vi "Page_Source_Initialize.vi"(8 "error in (no error)":errorcluster, 9 "ctlReferences":T1, 11 "AB_PackedLibrary in":refnum<class "AB_PackedLibrary.lvclass">) -> (0 "error out":errorcluster, 1 "supportedFunctions":T2, 3 "AB_PackedLibrary out":refnum<class "AB_PackedLibrary.lvclass">)   [LabVIEW 2020, in "AB_PackedLibrary.lvclass"]
uses:
  <vilib>/AppBuilder/AB_Classes/PackedLib/AB_PackedLibrary.lvclass
  <resource>/Framework/Providers/Builds/AppBuilder/AB_UI_Page_Source_Files_supportedFunctions.ctl
  <vilib>/AppBuilder/AB_Source_Inclusion.ctl
  <resource>/Framework/Providers/Builds/AppBuilder/AB_UI_Page_Source_Files_References.ctl
  <resource>/Framework/Providers/Common/provcom_StringGlobals.vi
  <vilib>/AppBuilder/AB_Classes/TargetFile/AB_Targetfile.lvclass
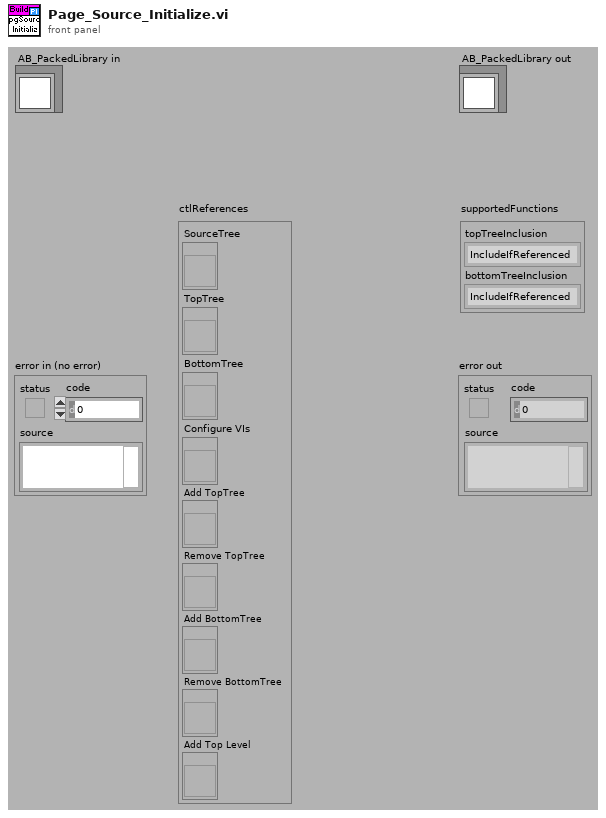
[diagram p1: front panel]
types:
  T1 = typedef "AB_UI_Page_Source_Files_References.ctl" = cluster{"SourceTree":refnum<vi>, "TopTree":refnum<vi>, "BottomTree":refnum<vi>, "Configure VIs":refnum<vi>, "Add TopTree":refnum<vi>, "Remove TopTree":refnum<vi>, "Add BottomTree":refnum<vi>, "Remove BottomTree":refnum<vi>, "Add Top Level":refnum<vi>}
  T2 = typedef "AB_UI_Page_Source_Files_supportedFunctions.ctl" = cluster{"topTreeInclusion":T3, "bottomTreeInclusion":T3}
  T3 = typedef "AB_Source_Inclusion.ctl" = enum16{"IncludeIfReferenced", "Include", "Exclude", "TopLevel"}
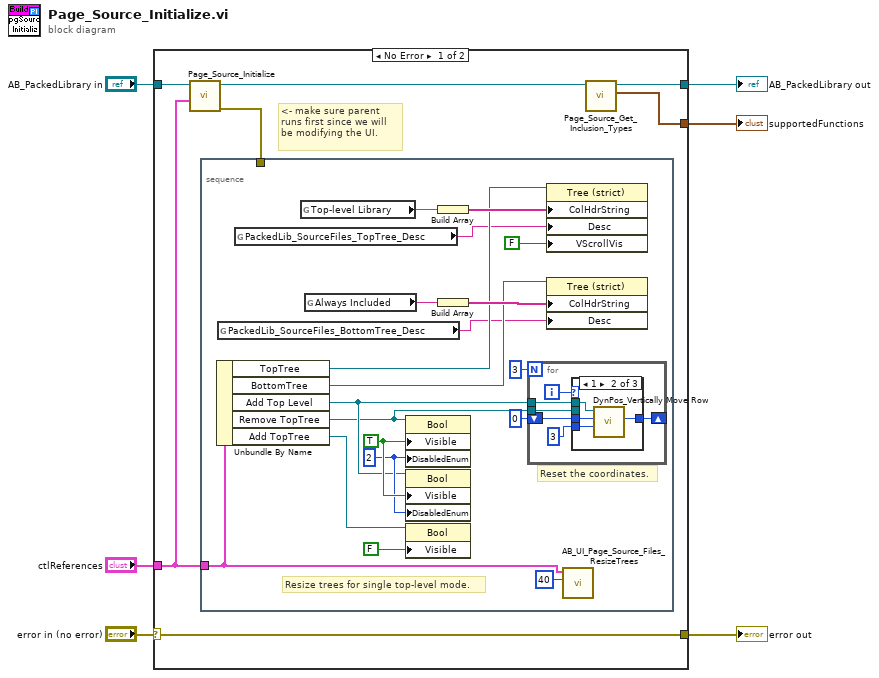
[diagram p0: block diagram]
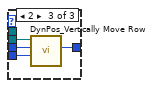
[diagram p3: hidden frame]
diagram:
  n1 = case shown="No Error" "error in (no error)" {
    selector: "error in (no error)" -> [w13 w49]
    tunnel: [w13 w49] -> w2
    tunnel: "AB_PackedLibrary in" -> [w10 w48]
    tunnel: "ctlReferences" -> [w8 _]
    tunnel: [w11 _] -> w3
    tunnel: [w12 w48] -> w1
    frame No Error {
      # "<- make sure parent runs first since we will be modifying the UI."
      n2 = call-parent "Page_Source_Initialize.vi"("ctlReferences"=w8, "AB_Build in"=w10) -> ("error out"=w7:errorcluster, "AB_Build out"=w9:refnum<class "AB_PackedLibrary.lvclass">)  [unwired: 7 in, 1 out]
      n3 = stacked-sequence {
        tunnel: w8 -> [w23]
        tunnel: w7 -> [_]
        frame #0 {
          w19 = 2
          w20 = TRUE ("Visible")
          # "Reset the coordinates."
          # "Resize trees for single top-level mode."
          n4 = Unbundle By Name(w23) -> ("TopTree"=w29:refnum<vi>, "BottomTree"=w28:refnum<vi>, "Add Top Level"=w16:refnum<vi>, "Remove TopTree"=w15:refnum<vi>, "Add TopTree"=w14:refnum<vi>)
          n5 = global read "provcom_StringGlobals.vi" "PackedLib_SourceFiles_BottomTree_Desc"() -> (w26:string)
          n6 = global read "provcom_StringGlobals.vi" "PackedLib_SourceFiles_TopTree_Desc"() -> (w27:string)
          n7 = global read "provcom_StringGlobals.vi" "Top-level Library"() -> (w25:string)
          n8 = global read "provcom_StringGlobals.vi" "Always Included"() -> (w32:string)
          n9 = property class="Bool"(reference=w15, "Visible"=w20, "DisabledEnum"=w19) -> ()  [unwired: 1 in, 2 out]
          n10 = property class="Bool"(reference=w16, "Visible"=w20, "DisabledEnum"=w19) -> ()  [unwired: 1 in, 2 out]
          n11 = property class="Bool"(reference=w14, "Visible"=FALSE) -> ()  [unwired: 1 in, 2 out]
          n12 = Build Array(w25) -> (w31:string[])
          n13 = Build Array(w32) -> (w30:string[])
          n14 = for {
            N: 3 -> [_]
            shift-right: [w35] -> _
            shift-left: 0 -> [w37]
            tunnel: w16 -> [w34]
            tunnel: w15 -> [w33]
            i -> [w38]
            n15 = case shown="1" w38 {
              tunnel: w37 -> [w39 w43 w47]
              tunnel: 3 -> [_ w42 w46]
              tunnel: [w39 w41 w45] -> w35
              tunnel: w34 -> [_ w40 _]
              tunnel: w33 -> [_ _ w44]
              frame 0, Default {
              }
              frame 1 {
                n16 = call <vilib>:"DynPos_Vertically Move Row.vi"("Pixel separation (6)"=w42, "Bottom of last control"=w43, "Control"=w40) -> ("Bottom pixel"=w41:i32)  [unwired: 7 in, 1 out]
              }
              frame 2 {
                n17 = call <vilib>:"DynPos_Vertically Move Row.vi"("Pixel separation (6)"=w46, "Bottom of last control"=w47, "Control"=w44) -> ("Bottom pixel"=w45:i32)  [unwired: 7 in, 1 out]
              }
            }
          }
          n18 = property class="Tree (strict)"(reference=w29, "ColHdrString"=w31, "Desc"=w27, "VScrollVis"=FALSE ("Visible Items:Vertical Scrollbar Visible")) -> ()  [unwired: 1 in, 2 out]
          n19 = property class="Tree (strict)"(reference=w28, "ColHdrString"=w30, "Desc"=w26) -> ()  [unwired: 1 in, 2 out]
          n20 = call <resource>:"AB_UI_Page_Source_Files_ResizeTrees.vi"("TopTree height"=40, "ctlReferences"=w23) -> ()  [unwired: 9 in, 1 out]
        }
      }
      n21 = call-dynamic "Page_Source_Get_Inclusion_Types.vi"("AB_PackedLibrary in"=w9) -> ("supportedFunctions"=w11:T2, "AB_PackedLibrary out"=w12:refnum<class "AB_PackedLibrary.lvclass">)  [unwired: 8 in, 1 out]
    }
    frame Error {
    }
  }
  "error out" <- w2
  "supportedFunctions" <- w3
  "AB_PackedLibrary out" <- w1
